vi "Error write to file.vi"(8 "error in (no error)":errorcluster, 11 "Description":string) -> ()   [LabVIEW 2013]
uses:
  ErrorCluster.ctl
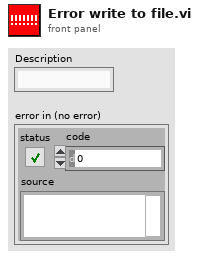
[diagram p1: front panel]
types:
  T1 = typedef "ErrorCluster.ctl" = cluster{"error out":errorcluster, "Description":string}
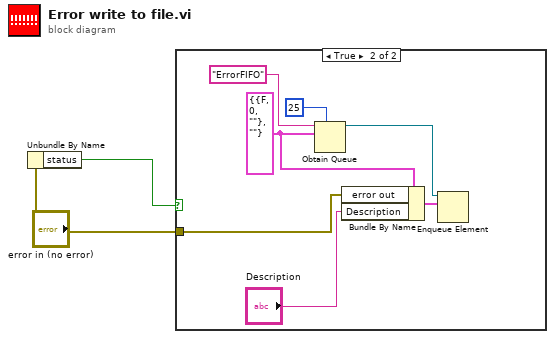
[diagram p0: block diagram]
diagram:
  n1 = Unbundle By Name("error in (no error)") -> ("status"=w2:bool)
  n2 = case shown="True" w2 {
    tunnel: "error in (no error)" -> [_ w4]
    frame False {
    }
    frame True {
      w7 = T1 {"error out"={"status"=FALSE, "code"=0, "source"=""}, "Description"=""} ("Cluster")
      n3 = Obtain Queue(max queue size (-1, unlimited)=25, name (unnamed)="ErrorFIFO", element data type=w7) -> (queue out=w6:refnum<queue>)  [unwired: 2 in, 2 out]
      n4 = Bundle By Name(cluster=w7, "error out"=w4, "Description"="Description") -> (w8:T1)
      n5 = Enqueue Element(queue=w6, element=w8) -> ()  [unwired: 2 in, 3 out]
    }
  }
